vi "PointAtGoalKeeperArea.vi"(9 "Field defense":dbl[](array[numeric]), 10 "IA State Input":T1, 11 "Array":dbl[](array[numeric])) -> (3 "Point inside goalkeeper area ?":bool)   [LabVIEW 2017]
uses:
  Core/AI Input.ctl
  Core/AI Robot.ctl
  Intel/Functions Enum.ctl
  Intel/AttackerStates.ctl
  Path Planning/RRT/PathDests.ctl
  Path Planning/RRT/PathDest.ctl
  Core/AI Ball.ctl
  Core/Field Size.ctl
  Core/AI Judge.ctl
  Intel/Command Enum.ctl
  Util/Events/Events.ctl
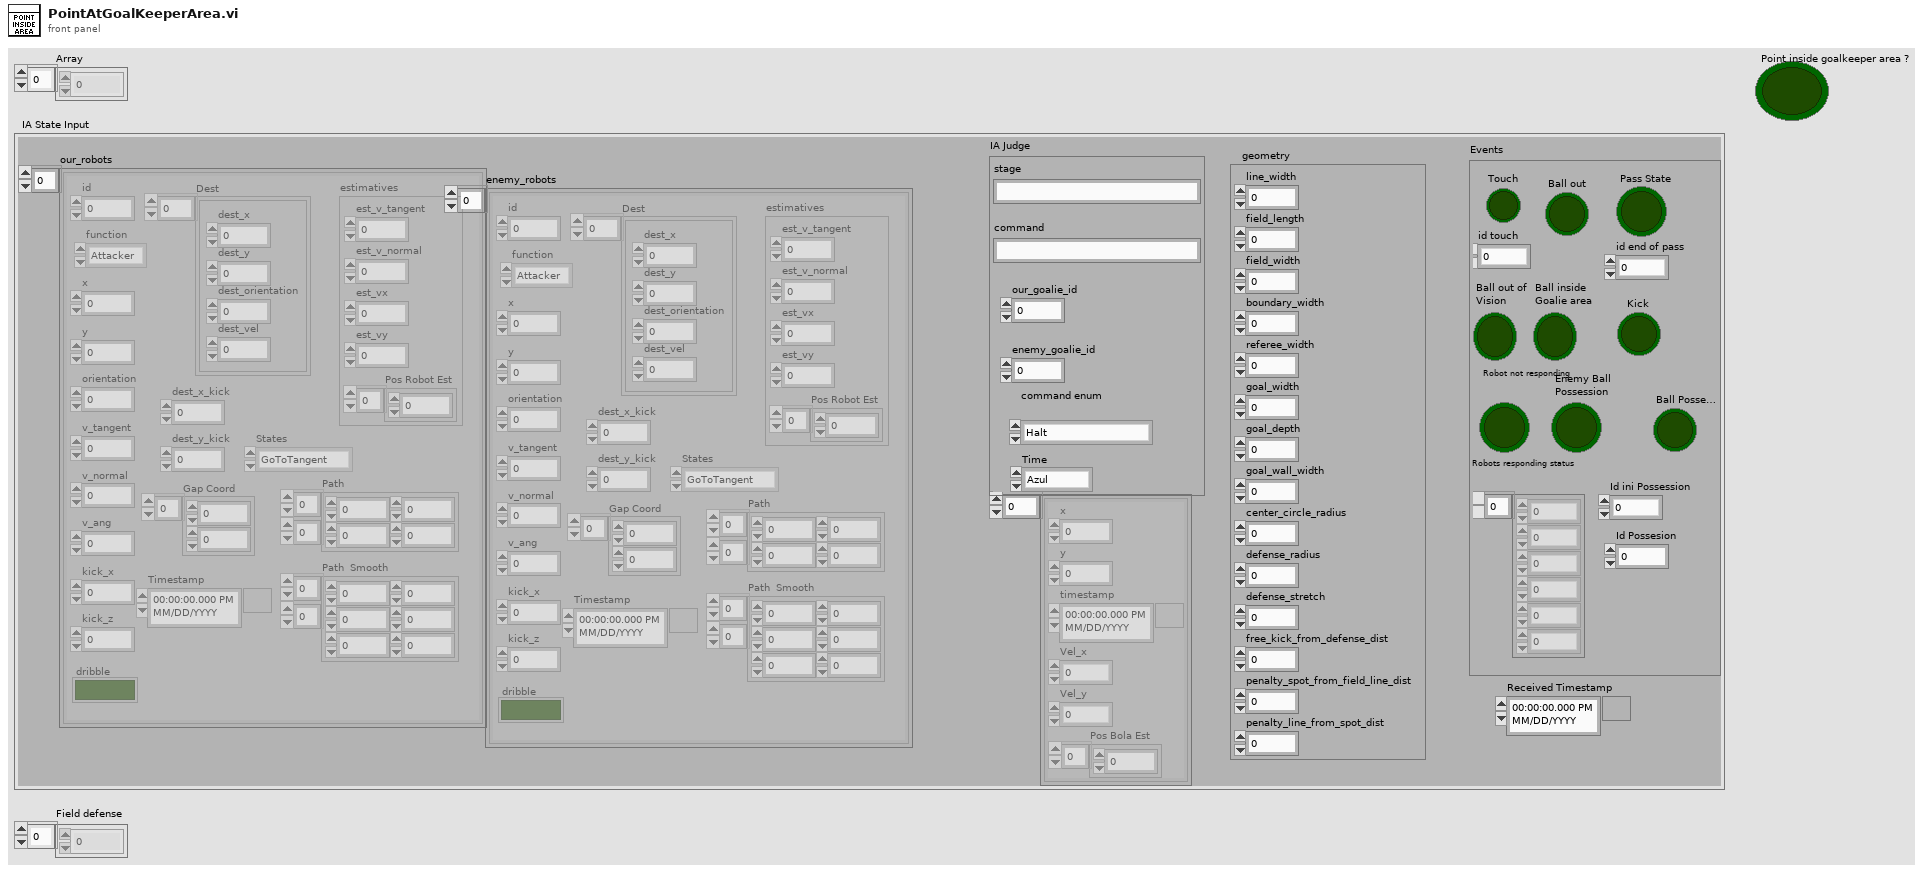
[diagram p1: front panel]
types:
  T1 = typedef "AI Input.ctl" = cluster{"our_robots":T2[], "enemy_robots":T2[], "balls":T7[], "geometry":T8, "IA Judge":T9, "Received Timestamp":timestamp, "Events":T11}
  T2 = typedef "AI Robot.ctl" = cluster{"id":u32, "function":T3, "x":dbl, "y":dbl, "orientation":dbl, "v_tangent":dbl, "v_normal":dbl, "v_ang":dbl, "kick_x":dbl, "kick_z":dbl, "dribble":bool, "Timestamp":timestamp, "estimatives":cluster{"est_v_tangent":dbl, "est_v_normal":dbl, "est_vx":dbl, "est_vy":dbl, "Pos Robot Est":dbl[]}, "dest_x_kick":dbl, "dest_y_kick":dbl, "Gap Coord":dbl[], "States":T4, "Path ":dbl[][], "Path  Smooth":dbl[][], "Dest":T5}
  T3 = typedef "Functions Enum.ctl" = enum16{"Attacker", "Goalie", "Defender", "Striker", "Goto 0", "Dummy", "Kicker", "ZigZag"}
  T4 = typedef "AttackerStates.ctl" = enum16{"Pass", "GoToTangent", "BallGetting", "GoToKick", ""}
  T5 = typedef "PathDests.ctl" = T6[]
  T6 = typedef "PathDest.ctl" = cluster{"dest_x":dbl, "dest_y":dbl, "dest_orientation":dbl, "dest_vel":dbl}
  T7 = typedef "AI Ball.ctl" = cluster{"x":dbl, "y":dbl, "timestamp":timestamp, "Vel_x":dbl, "Vel_y":dbl, "Pos Bola Est":dbl[]}
  T8 = typedef "Field Size.ctl" = cluster{"line_width":u32, "field_length":u32, "field_width":u32, "boundary_width":u32, "referee_width":u32, "goal_width":u32, "goal_depth":u32, "goal_wall_width":u32, "center_circle_radius":u32, "defense_radius":u32, "defense_stretch":u32, "free_kick_from_defense_dist":u32, "penalty_spot_from_field_line_dist":u32, "penalty_line_from_spot_dist":u32}
  T9 = typedef "AI Judge.ctl" = cluster{"stage":string, "command":string, "our_goalie_id":dbl, "enemy_goalie_id":dbl, "command enum":T10, "Time":enum16{"Azul", "Amarelo"}}
  T10 = typedef "Command Enum.ctl" = enum16{"Halt", "Stop", "Force Start", "PKA Normal Start", "Prepare Kickoff Ally", "PKE Normal Start", "Prepare Kickoff Enemy", "Prepare Penalty Ally", "PPA Normal Start", "Prepare Penalty Enemy", "PPE Normal Start", "Direct Free Enemy", "Direct Free Ally", "Indirect Free Enemy", "Indirect Free Ally", "Timeout Enemy", "Timeout Ally", "Goal Enemy", "Goal Ally", "Ball Placement Enemy", "Ball Placement Ally", "Normal Half Time", "Extra Time Break", "Extra Half Time", "None", "Post Game"}
  T11 = typedef "Events.ctl" = cluster{"Touch":bool, "Ball out":bool, "id touch":dbl, "Ball out of \nVision":bool, "Ball inside \nGoalie area":bool, "Robot not responding":bool, "Robots responding status":dbl[], "Enemy Ball \nPossession":bool, "Pass State":bool, "id end of pass":dbl, "Kick":bool, "Id ini Possession":dbl, "Ball Possesion":bool, "Id Possesion":dbl}
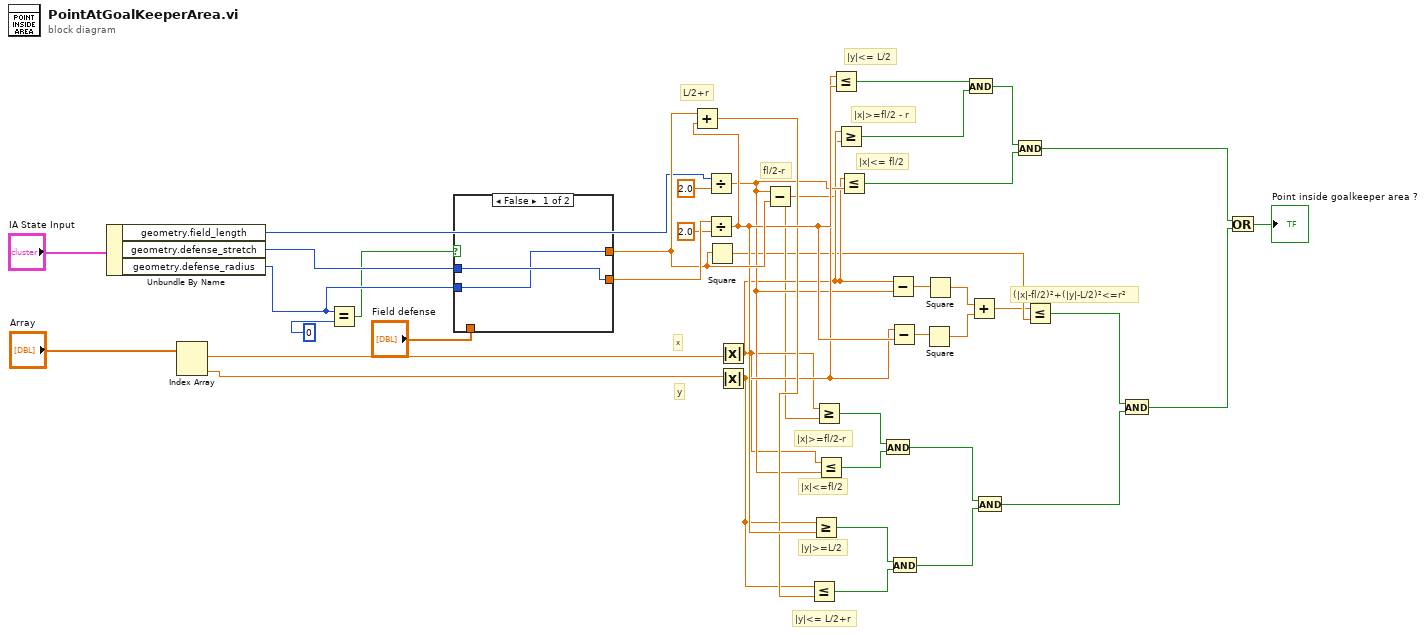
[diagram p0: block diagram]
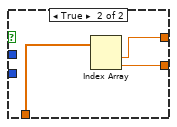
[diagram p2: hidden frame]
diagram:
  # "y"
  # "x"
  # "|y|<= L/2+r"
  # "L/2+r"
  # "|y|>=L/2"
  # "|x|<=fl/2"
  # "|x|>=fl/2-r"
  # "fl/2-r"
  # "(|x|-fl/2)²+(|y|-L/2)²<=r²"
  # "|x|<= fl/2"
  # "|x|>=fl/2 - r"
  # "|y|<= L/2"
  n1 = Unbundle By Name("IA State Input") -> ("geometry.field_length"=w3:u32, "geometry.defense_stretch"=w36:u32, "geometry.defense_radius"=w37:u32)
  n2 = Index Array(array="Array") -> (element #1=w40:dbl, element #2=w41:dbl)  [unwired: 2 in]
  n3 = Equal?(x=w37, y=u32 0) -> (x = y?=w33:bool)
  n4 = case shown="False" w33 {
    tunnel: [w42 w46] -> w34
    tunnel: [w43 w45] -> w35
    tunnel: "Field defense" -> [_ w44]
    tunnel: w36 -> [w43 _]
    tunnel: w37 -> [w42 _]
    frame False {
    }
    frame True {
      n5 = Index Array(array=w44) -> (element #1=w46:dbl, element #2=w45:dbl)  [unwired: 2 in]
    }
  }
  n6 = Divide(x=w3, y=2.0) -> (x/y=w18:dbl)
  n7 = Divide(x=w35, y=2.0) -> (x/y=w30:dbl)
  n8 = Add(x=w34, y=w30) -> (x+y=w20:dbl)
  n9 = Square(x=w34) -> (x^2=w13:dbl)
  n10 = Absolute Value(x=w40) -> (abs(x)=w15:dbl)
  n11 = Absolute Value(x=w41) -> (abs(x)=w19:dbl)
  n12 = Subtract(x=w18, y=w34) -> (x-y=w14:dbl)
  n13 = Less Or Equal?(x=w19, y=w20) -> (x <= y?=w22:bool)
  n14 = Greater Or Equal?(x=w19, y=w30) -> (x >= y?=w21:bool)
  n15 = Greater Or Equal?(x=w15, y=w14) -> (x >= y?=w16:bool)
  n16 = Less Or Equal?(x=w15, y=w18) -> (x <= y?=w17:bool)
  n17 = Less Or Equal?(x=w19, y=w30) -> (x <= y?=w4:bool)
  n18 = Greater Or Equal?(x=w15, y=w14) -> (x >= y?=w5:bool)
  n19 = Less Or Equal?(x=w15, y=w18) -> (x <= y?=w7:bool)
  n20 = And(x=w16, y=w17) -> (x .and. y?=w23:bool)
  n21 = Subtract(x=w15, y=w18) -> (x-y=w8:dbl)
  n22 = Subtract(x=w19, y=w30) -> (x-y=w9:dbl)
  n23 = And(x=w21, y=w22) -> (x .and. y?=w24:bool)
  n24 = Square(x=w9) -> (x^2=w11:dbl)
  n25 = Square(x=w8) -> (x^2=w10:dbl)
  n26 = And(x=w4, y=w5) -> (x .and. y?=w6:bool)
  n27 = Add(x=w10, y=w11) -> (x+y=w12:dbl)
  n28 = And(x=w23, y=w24) -> (x .and. y?=w26:bool)
  n29 = And(x=w6, y=w7) -> (x .and. y?=w27:bool)
  n30 = Less Or Equal?(x=w12, y=w13) -> (x <= y?=w25:bool)
  n31 = And(x=w25, y=w26) -> (x .and. y?=w28:bool)
  n32 = Or(x=w27, y=w28) -> (x .or. y?=→"Point inside goalkeeper area ?":bool)
